vi "Untitled 2.vi"(0 "TTL TRIG_(0) Delay":dbl=0.1, 1 "TTL TRIG_(0) Width":dbl=0.2, 5 "Stop (F)":bool, 7 "error in":errorcluster) -> (20 "Image Out":T1(plugin-control), 26 "Stopped":bool, 27 "error out":errorcluster)   [LabVIEW 2015]
doc: "Creates, and edits acquisitions using the NI Vision Acquisition Express VI.\n\nThe NI Vision Acquisition Wizard is launched by placing the Express VI on the block diagram. Select an acquisition source and configure an acquisition using NI-IMAQ, NI-IMAQdx, or simulate an acquisition by reading an AVI or image files from a folder. After an acquisition is configured, select controls and indicators to be able to programmatically set in LabVIEW. Double-click the Vision Acquisition Express VI to edit the acquisition.\n\nNote: Any images created by the Express VI need to be disposed after use. Use the IMAQ Dispose.vi to cleanup the images output by the Express VI when they are no longer needed."
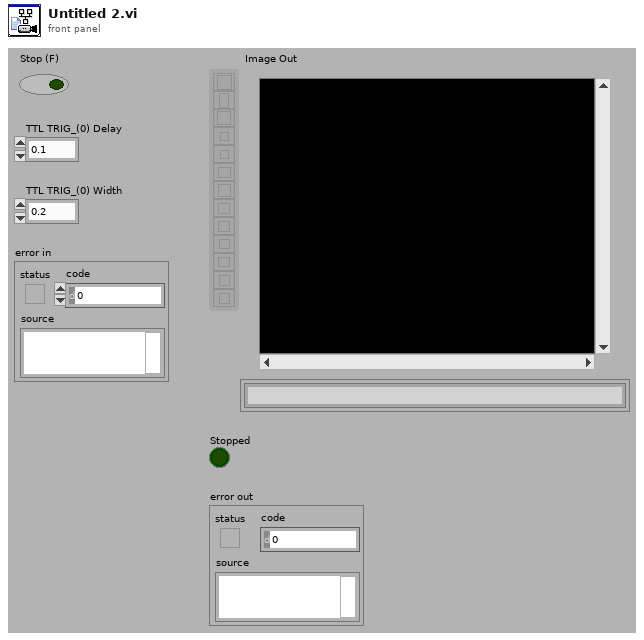
[diagram p1: front panel]
types:
  T1 = typedef "IMAQ Image.ctl" = refnum<image>
  T2 = cluster{"TTL TRIG_(0) Delay":dbl, "TTL TRIG_(0) Width":dbl, "Pulse Polarity":enum16{"High True ", "Low True"}, "Units":enum16{"Seconds", "Scaled Encoder Counts"}}
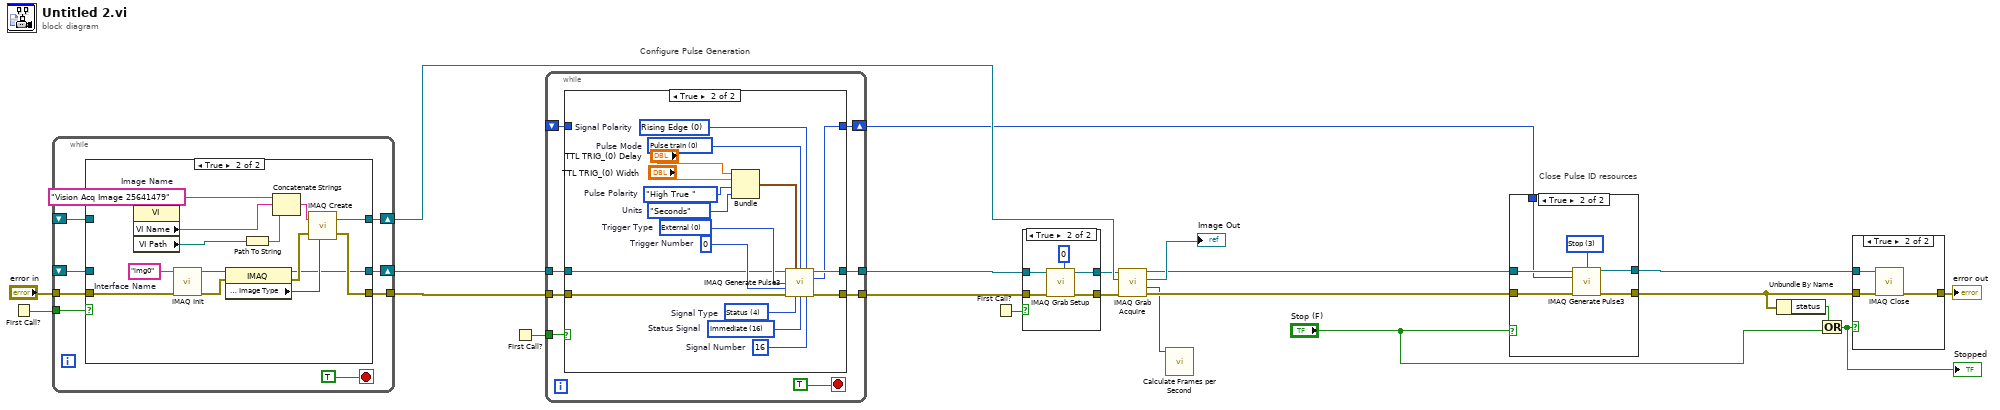
[diagram p0: block diagram]
diagram:
  # "Close Pulse ID resources"
  # "Configure Pulse Generation"
  n1 = First Call?() -> (First Call?: T/F=w22:bool)
  n2 = while "While Loop_template0_template1" {
    tunnel: w22 -> [w30]
    tunnel: [w27] -> w20
    tunnel: "error in" -> [w26]
    shift-right: [w24] -> w15
    shift-left: _ -> [w23]
    shift-right: [w29] -> w18
    shift-left: _ -> [w28]
    stop <- TRUE ("_template0_template1") stop-if-true
    n3 = case "Case Structure_template0_template1" shown="True" w30 {
      tunnel: [w33 w34] -> w29
      tunnel: w28 -> [w33 _]
      tunnel: [w32 w35] -> w27
      tunnel: w26 -> [w32 w43]
      tunnel: [w31 w45] -> w24
      tunnel: w23 -> [w31 _]
      frame False {
      }
      frame True {
        w44 = "img0"  # Interface Name
        w39 = "Vision Acq Image 25641479"  # Image Name
        n4 = property class="VI"() -> ("VI Name"=w41:string, "VI Path"=w42:path)  [unwired: 2 in, 2 out]
        n5 = call <vilib>:"IMAQ Init.vi"("error in (no error)"=w43, "Interface Name"=w44) -> ("error out"=w36:errorcluster, "IMAQ Session Out"=w37:refnum<k11>)  [unwired: 8 out]
        n6 = property class="IMAQ"(reference=w37, error in=w36) -> (reference out=w34:refnum<k11>, error out=w47:errorcluster, "Image Parameters : Image Type"=w46:u32)
        n7 = Path To String(path=w42) -> (string=w40:string)
        n8 = Concatenate Strings(w39, w41, w40) -> (w38:string)
        n9 = call "IMAQ Create"("Image Name"=w38, "Image Type"=w46, "error in (no error)"=w47) -> ("New Image"=w45:T1, "error out"=w35:errorcluster)  [unwired: 1 in, 1 out]
      }
    }
  }
  n10 = First Call?() -> (First Call?: T/F=w19:bool)
  n11 = while {
    tunnel: w19 -> [w55]
    tunnel: w18 -> [w54]
    tunnel: [w53] -> w13
    tunnel: [w52] -> w17
    tunnel: w20 -> [w51]
    shift-right: [w50] -> w6
    shift-left: _ -> [w48]
    stop <- TRUE stop-if-true
    n12 = case "Case Structure_template0_template1" shown="True" w55 {
      tunnel: w54 -> [w58 w63]
      tunnel: w51 -> [w57 w60]
      tunnel: [w58 w62] -> w53
      tunnel: [w57 w61] -> w52
      tunnel: [w56 w59] -> w50
      tunnel: w48 -> [w56 _]
      frame False {
      }
      frame True {
        w68 = enum16{"High True ", "Low True"}."High True "  # Pulse Polarity
        w69 = enum16{"Seconds", "Scaled Encoder Counts"}."Seconds"  # Units
        w64 = u32 0 items=["Rising Edge", "Falling Edge"]  # Signal Polarity
        w72 = u32 0  # Trigger Number
        w71 = u32 0 items=["External"=0, "RTSI"=1, "ISO Out"=3]  # Trigger Type
        w75 = u32 16  # Signal Number
        w74 = u32 16 items=["Acquisition in progress"=15, "Acquisition done"=8, "Horizontal Synchronization Signal"=18, "Vertical Synchronization Signal"=19, "Frame start"=9, "Frame done"=10, "Immediate"=16]  # Status Signal
        w73 = u32 4 items=["External"=0, "RTSI "=1, "ISO In"=2, "Status"=4]  # Signal Type
        w65 = u32 0 items=["Pulse train", "Single pulse", "Rearmed pulse", "Stop"]  # Pulse Mode
        n13 = Bundle("TTL TRIG_(0) Delay"="TTL TRIG_(0) Delay", "TTL TRIG_(0) Width"="TTL TRIG_(0) Width", "Pulse Polarity"=w68, "Units"=w69) -> (w70:T2)  [unwired: 1 out]
        n14 = call <vilib>:"IMAQ Generate Pulse3.vi"("IMAQ Session In"=w63, "Pulse Parameters"=w70, "Pulse Mode"=w65, "Signal polarity"=w64, "Trigger Type"=w71, "Trigger Number"=w72, "error in (no error)"=w60, "Signal Type"=w73, "Status Signal"=w74, "Signal Number"=w75) -> ("IMAQ Session Out"=w62:refnum<k11>, "Pulse ID Out"=w59:u32, "error out"=w61:errorcluster)  [unwired: 1 in, 2 out]
      }
    }
  }
  n15 = First Call?() -> (First Call?: T/F=w12:bool)
  n16 = case shown="True" w12 {
    tunnel: w13 -> [w77 w81]
    tunnel: w17 -> [w76 w80]
    tunnel: [w77 w79] -> w11
    tunnel: [w76 w78] -> w10
    frame False {
    }
    frame True {
      n17 = call <vilib>:"IMAQ Grab Setup.vi"("Channel"=0, "error in (no error)"=w80, "IMAQ Session In"=w81) -> ("error out"=w78:errorcluster, "IMAQ Session Out"=w79:refnum<k11>)  [unwired: 7 out]
    }
  }
  n18 = call <vilib>:"IMAQ Grab Acquire.vi"("error in (no error)"=w10, "Image In"=w15, "IMAQ Session In"=w11) -> ("error out"=w14:errorcluster, "Acquired Buffer Number"=w9:u32, "Image Out"=→"Image Out":T1, "IMAQ Session Out"=w7:refnum<k11>)  [unwired: 1 in, 4 out]
  n19 = call <vilib>:"Calculate Frames per Second.vi"("Buffer Number"=w9) -> ()  [unwired: 2 in, 9 out]
  n20 = case shown="True" "Stop (F)" {
    tunnel: [w84 w90] -> w5
    tunnel: [w83 w89] -> w8
    tunnel: w14 -> [w83 w88]
    tunnel: w7 -> [w84 w87]
    tunnel: w6 -> [_ w86]
    frame False {
    }
    frame True {
      w85 = u32 3 items=["Pulse train", "Single pulse", "Rearmed pulse", "Stop"] ("Pulse Mode")
      n21 = call <vilib>:"IMAQ Generate Pulse3.vi"("IMAQ Session In"=w87, "Pulse Mode"=w85, "Pulse ID In"=w86, "error in (no error)"=w88) -> ("IMAQ Session Out"=w90:refnum<k11>, "error out"=w89:errorcluster)  [unwired: 7 in, 3 out]
    }
  }
  n22 = Unbundle By Name(w8) -> ("status"=w2:bool)
  n23 = Or(x=w2, y="Stop (F)") -> (x .or. y?=w1:bool)
  "Stopped" <- w1
  n24 = case "Case Structure_template2" shown="True" w1 {
    tunnel: [w91 w94] -> w4
    tunnel: w5 -> [_ w92]
    tunnel: w8 -> [w91 w93]
    frame False {
    }
    frame True {
      n25 = call <vilib>:"IMAQ Close.vi"("error in (no error)"=w93, "IMAQ Session In"=w92) -> ("error out"=w94:errorcluster)  [unwired: 9 out]
    }
  }
  "error out" <- w4
